vi "niScope Fetch Measurement Stats.vi"(0 "instrument handle":refnum<k15>, 1 "timeout":dbl=5.0 format="%.2f", 5 "channels":string="0", 7 "scalar measurement":T2=4000 items=["None"=4000, "Frequency"=2, "Average Frequency"=1016, "FFT Frequency"=1008, "Period"=3, "Average Period"=1015, "Rise Time"=0, "Fall Time"=1, "Rising Slew Rate"=1010, "Falling Slew Rate"=1011, "Overshoot"=18, "Preshoot"=19, "Voltage RMS"=4, "Voltage Cycle RMS"=16, "AC Estimate"=1012, "FFT Amplitude"=1009, "Voltage Average"=10, "Voltage Cycle Average"=17, "DC Estimate"=1013, "Voltage Max"=6, "Voltage Min"=7, "Voltage Peak-to-Peak"=5, "Voltage High"=8, "Voltage Low"=9, "Voltage Amplitude"=15, "Voltage Top"=1007, "Voltage Base"=1006, "Voltage Base-to-Top"=1017, "Negative Width"=11, "Positive Width"=12, "Negative Duty Cycle"=13, "Positive Duty Cycle"=14, "Integral"=1005, "Area"=1003, "Cycle Area"=1004, "Time Delay"=1014, "Phase Delay"=1018, "Low Ref Volts"=1000, "Mid Ref Volts"=1001, "High Ref Volts"=1002, "Volt. Hist. Mean"=2000, "Volt. Hist. Stdev"=2001, "Volt. Hist. Median"=2003, "Volt. Hist. Mode"=2010, "Volt. Hist. Max"=2005, "Volt. Hist. Min"=2006, "Volt. Hist. Peak-to-Peak"=2002, "Volt. Hist. Mean + Stdev"=2007, "Volt. Hist. Mean + 2 Stdev"=2008, "Volt. Hist. Mean + 3 Stdev"=2009, "Volt. Hist. Hits"=2004, "Volt. Hist. New Hits"=2011, "Time Hist. Mean"=3000, "Time Hist. Stdev"=3001, "Time Hist. Median"=3003, "Time Hist. Mode"=3010, "Time Hist. Max"=3005, "Time Hist. Min"=3006, "Time Hist. Peak-to-Peak"=3002, "Time Hist. Mean + Stdev"=3007, "Time Hist. Mean + 2 Stdev"=3008, "Time Hist. Mean + 3 Stdev"=3009, "Time Hist. Hits"=3004, "Time Hist. New Hits"=3011], 11 "error in":errorcluster) -> (4 "instrument handle out":refnum<k15>, 6 "stats":T1 {"max" format="%^.2e"; "min" format="%^.2e"; "stdev" format="%^.2e"; "mean" format="%^.2e"; "result" format="%^.2e"}, 15 "error out":errorcluster)   [LabVIEW 2013]
doc: "Obtains a waveform measurement and returns the measurement value for a single channel and record. Specify a particular measurement type, such as rise time, frequency, or voltage peak-to-peak. The waveform on which the digitizer calculates the waveform measurement is from an acquisition that you previously initiated. The statistics for the specified measurement are also returned, where the statistics are updated once every acquisition when the specified measurement is fetched by any of the Fetch/Read measurement VIs."
uses:
  <instrlib>/niScope/Controls/niScope scalar measurement.ctl
  niScope_32.dll
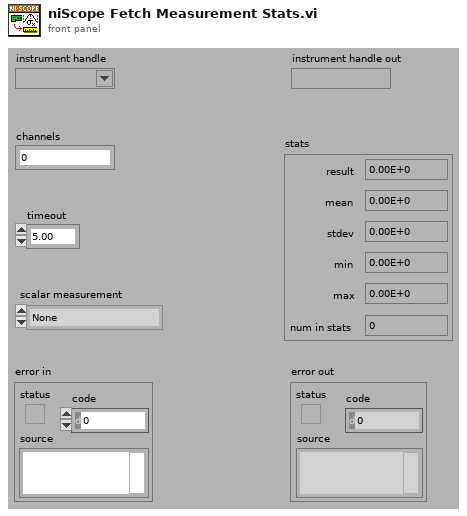
[diagram p1: front panel]
types:
  T1 = cluster{"result":dbl, "mean":dbl, "stdev":dbl, "min":dbl, "max":dbl, "num in stats":i32}
  T2 = typedef "niScope scalar measurement.ctl" = i32
  T3 = cluster{"result":dbl, "mean":dbl, "stdev":dbl, "min":dbl, "max":dbl, "numInStats":i32}
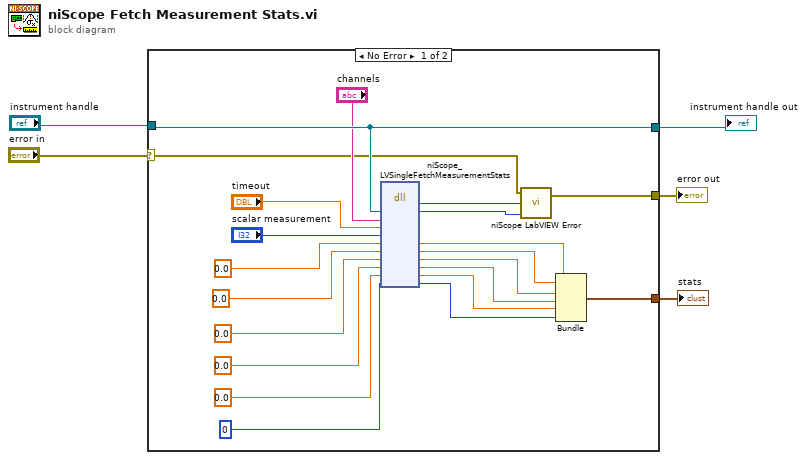
[diagram p0: block diagram]
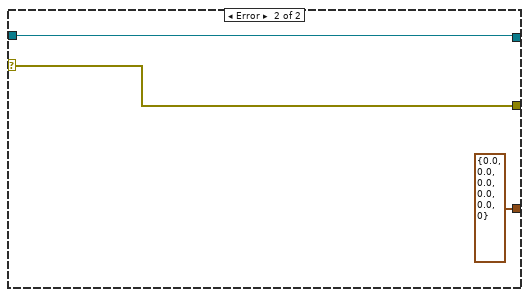
[diagram p2: hidden frame]
diagram:
  n1 = case shown="No Error" "error in" {
    selector: "error in" -> [w6 w27]
    tunnel: [w26 w27] -> w5
    tunnel: "instrument handle" -> [w23 w29]
    tunnel: [w23 w29] -> w4
    tunnel: [w13 T3 {"result"=0.0, "mean"=0.0, "stdev"=0.0, "min"=0.0, "max"=0.0, "numInStats"=0}] -> w2
    frame No Error {
      n2 = dll-call lib="niScope_*.*" fn="niScope_LVSingleFetchMeasurementStats"("instrument handle"=w23, "channel"="channels", "timeout"="timeout", "scalarMeasFunction"="scalar measurement", "result"=0.0, "mean"=0.0, "stdev"=0.0, "min"=0.0, "max"=0.0, "numInStats"=0) -> ("status"=w25:i32, "instrument handle"=w24:u32, "result"=w19:dbl, "mean"=w18:dbl, "stdev"=w17:dbl, "min"=w16:dbl, "max"=w15:dbl, "numInStats"=w14:i32)  [unwired: 6 in, 2 out]
      n3 = call <instrlib>:"niScope LabVIEW Error.vi"("instrument handle"=w24, "niScope error code (0)"=w25, "error in (no error)"=w6) -> ("error out"=w26:errorcluster)  [unwired: 2 in]
      n4 = Bundle("result"=w19, "mean"=w18, "stdev"=w17, "min"=w16, "max"=w15, "numInStats"=w14) -> (w13:T3)  [unwired: 1 in]
    }
    frame Error {
    }
  }
  "instrument handle out" <- w4
  "error out" <- w5
  "stats" <- w2
